vi "for final test.vi"() -> ()   [LabVIEW 2015]
panel:
  in  "Array 3":i32[][](array[numeric])
  out "Array 2":bool[](array[boolean])
  out "Array":string[](array[string])
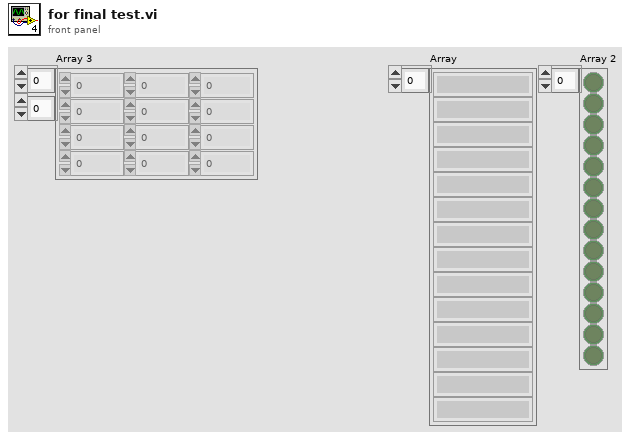
[diagram p1: front panel]
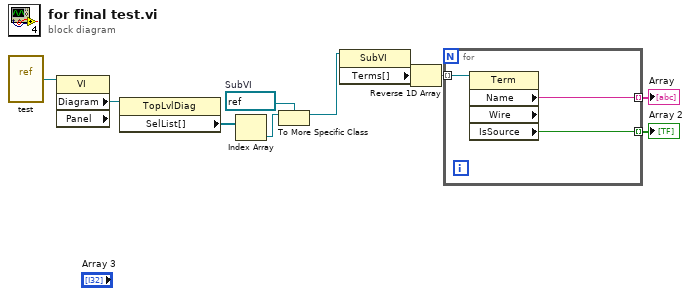
[diagram p0: block diagram]
diagram:
  w6 = refnum<vi> refnum  # SubVI
  n1 = vi-ref "test.vi"() -> (w9:refnum<vi>)
  n2 = property class="VI" props=["Diagram", "Panel"](reference=w9) -> ("Diagram"=w10:refnum<vi>)  [unwired: 1 in, 3 out]
  n3 = property class="TopLvlDiag"(reference=w10) -> ("SelList[]"=w8:refnum<vi>[])  [unwired: 1 in, 2 out]
  n4 = Index Array(array=w8) -> (element=w7:refnum<vi>)  [unwired: 1 in]
  n5 = To More Specific Class(target class=w6, reference=w7) -> (specific class reference=w5:refnum<vi>)  [unwired: 1 in, 1 out]
  n6 = property class="SubVI"(reference=w5) -> ("Terms[]"=w4:refnum<vi>[])  [unwired: 1 in, 2 out]
  n7 = Reverse 1D Array(array=w4) -> (reversed array=w1:refnum<vi>[])
  n8 = for {
    tunnel: w1 -> [w13] mode=indexing
    tunnel: [w12] -> w3 mode=indexing
    tunnel: [w11] -> w2 mode=indexing
    n9 = property class="Term" props=["Name", "Wire", "IsSource"](reference=w13) -> ("Name"=w12:string, "IsSource"=w11:bool)  [unwired: 1 in, 3 out]
  }
  "Array" <- w3
  "Array 2" <- w2
